vi "Linear Brass25 Calculations.vi"(0 "Power":dbl, 2 "Diameter":dbl, 3 "X1":dbl[](array[numeric]), 5 "T1":dbl[](array[numeric]), 6 "X2":dbl[](array[numeric]), 10 "T2":dbl[](array[numeric]), 11 "X3":dbl[](array[numeric]), 12 "T3":dbl[](array[numeric])) -> (16 "K1-2":dbl, 17 "K2-3":dbl, 18 "K3-4":dbl, 19 "K4-5":dbl, 20 "XY Graph":cluster{"Ramp Pattern":dbl[], dbl[]}[](graph), 21 "K5-6":dbl, 22 "K6-7":dbl, 23 "K7-8":dbl)   [LabVIEW 2017]
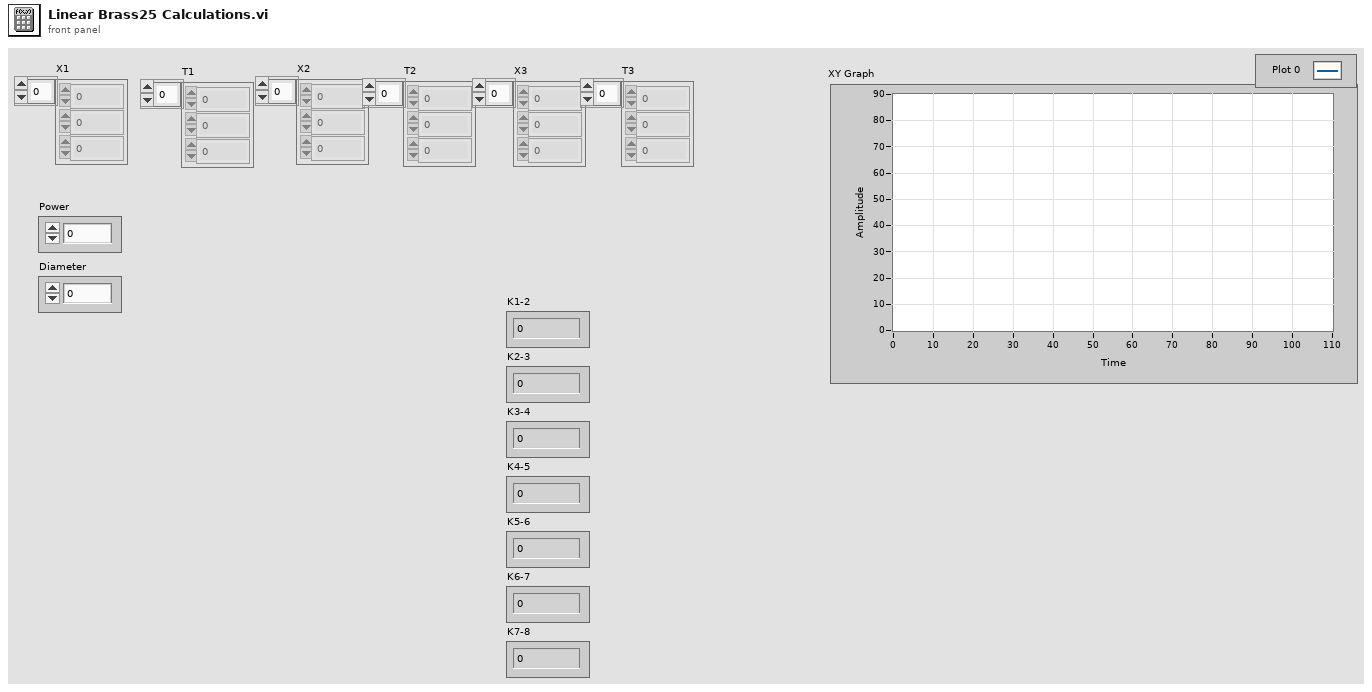
[diagram p1: front panel]
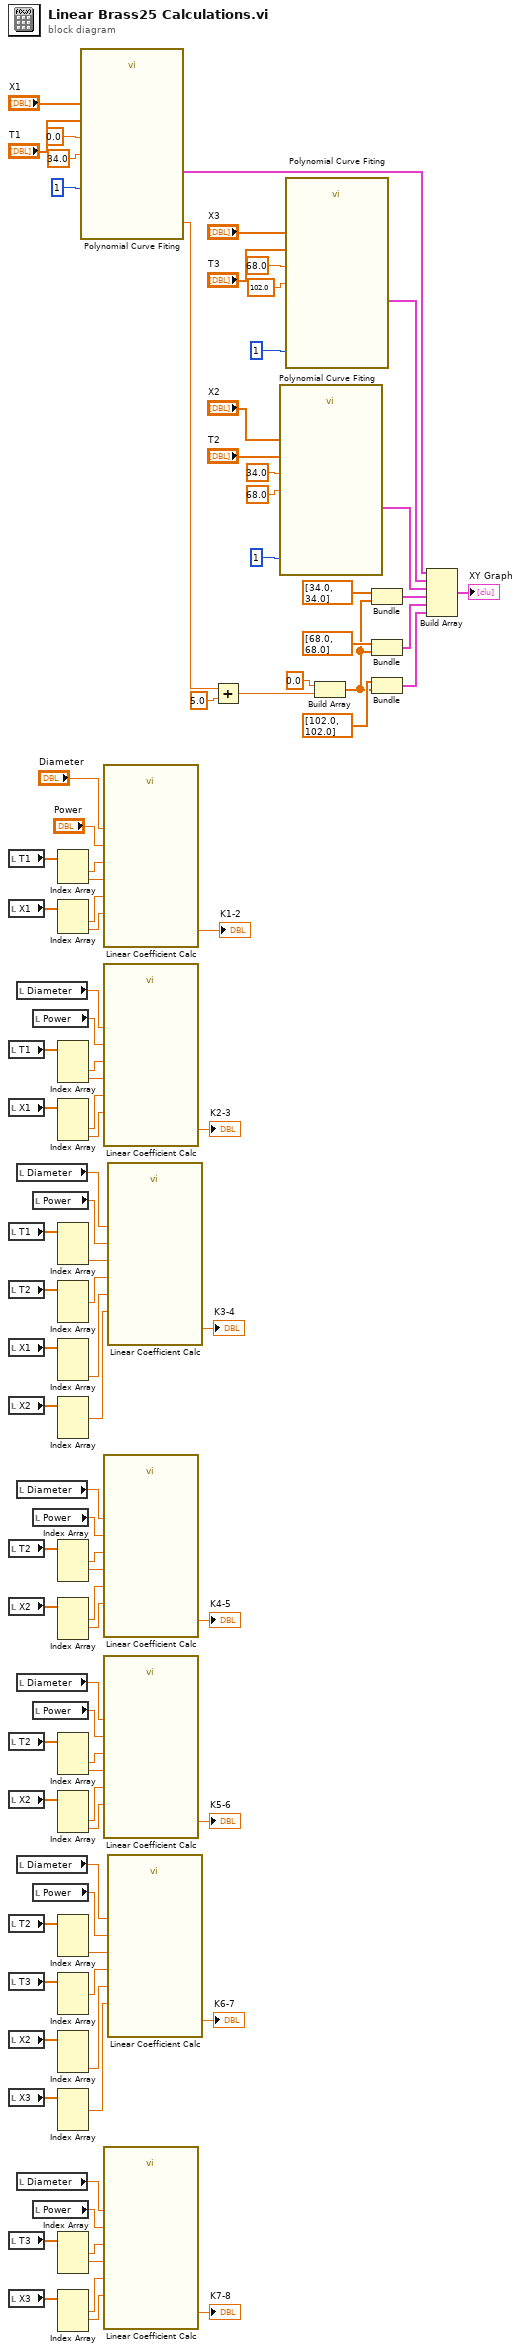
[diagram p0: block diagram]
diagram:
  n1 = local read "T1"() -> (w65:dbl[])
  n2 = local read "X1"() -> (w64:dbl[])
  n3 = local read "T1"() -> (w56:dbl[])
  n4 = local read "X1"() -> (w57:dbl[])
  n5 = local read "T1"() -> (w49:dbl[])
  n6 = local read "T2"() -> (w43:dbl[])
  n7 = local read "X1"() -> (w48:dbl[])
  n8 = local read "X2"() -> (w41:dbl[])
  n9 = local read "T2"() -> (w11:dbl[])
  n10 = local read "X2"() -> (w12:dbl[])
  n11 = local read "T2"() -> (w34:dbl[])
  n12 = local read "X2"() -> (w33:dbl[])
  n13 = local read "T2"() -> (w21:dbl[])
  n14 = local read "T3"() -> (w27:dbl[])
  n15 = local read "X2"() -> (w22:dbl[])
  n16 = local read "X3"() -> (w29:dbl[])
  n17 = local read "T3"() -> (w16:dbl[])
  n18 = local read "X3"() -> (w17:dbl[])
  n19 = local read "Diameter"() -> (w60:dbl)
  n20 = local read "Diameter"() -> (w46:dbl)
  n21 = local read "Diameter"() -> (w14:dbl)
  n22 = local read "Diameter"() -> (w31:dbl)
  n23 = local read "Diameter"() -> (w24:dbl)
  n24 = local read "Diameter"() -> (w19:dbl)
  n25 = local read "Power"() -> (w59:dbl)
  n26 = local read "Power"() -> (w47:dbl)
  n27 = local read "Power"() -> (w13:dbl)
  n28 = local read "Power"() -> (w32:dbl)
  n29 = local read "Power"() -> (w23:dbl)
  n30 = local read "Power"() -> (w18:dbl)
  n31 = Index Array(array=w65) -> (element #1=w63:dbl, element #2=w62:dbl)  [unwired: 2 in]
  n32 = Index Array(array=w64) -> (element #1=w61:dbl, element #2=w58:dbl)  [unwired: 2 in]
  n33 = Index Array(array=w56) -> (element #2=w55:dbl, element #3=w54:dbl)  [unwired: 3 in, 1 out]
  n34 = Index Array(array=w57) -> (element #2=w53:dbl, element #3=w52:dbl)  [unwired: 3 in, 1 out]
  n35 = Index Array(array=w49) -> (element #3=w45:dbl)  [unwired: 3 in, 2 out]
  n36 = Index Array(array=w43) -> (element #1=w42:dbl)  [unwired: 3 in, 2 out]
  n37 = Index Array(array=w48) -> (element #3=w44:dbl)  [unwired: 3 in, 2 out]
  n38 = Index Array(array=w41) -> (element #1=w40:dbl)  [unwired: 3 in, 2 out]
  n39 = Index Array(array=w11) -> (element #1=w9:dbl, element #2=w8:dbl)  [unwired: 3 in, 1 out]
  n40 = Index Array(array=w12) -> (element #1=w7:dbl, element #2=w6:dbl)  [unwired: 3 in, 1 out]
  n41 = Index Array(array=w34) -> (element #2=w35:dbl, element #3=w36:dbl)  [unwired: 3 in, 1 out]
  n42 = Index Array(array=w33) -> (element #2=w37:dbl, element #3=w38:dbl)  [unwired: 3 in, 1 out]
  n43 = Index Array(array=w21) -> (element #3=w25:dbl)  [unwired: 3 in, 2 out]
  n44 = Index Array(array=w27) -> (element #1=w28:dbl)  [unwired: 3 in, 2 out]
  n45 = Index Array(array=w22) -> (element #3=w26:dbl)  [unwired: 3 in, 2 out]
  n46 = Index Array(array=w29) -> (element #1=w30:dbl)  [unwired: 3 in, 2 out]
  n47 = Index Array(array=w16) -> (element #1=w5:dbl, element #2=w4:dbl)  [unwired: 3 in, 1 out]
  n48 = Index Array(array=w17) -> (element #1=w3:dbl, element #2=w2:dbl)  [unwired: 3 in, 1 out]
  n49 = call "Polynomial Curve Fiting.vi"("polynomial order"=1, "end"=34.0, "start"=0.0, "Y"="T1", "X"="X1") -> ("T First"=w71:dbl, "XY Graph"=w83:cluster{"Ramp Pattern":dbl[], dbl[]})  [unwired: 1 out]
  n50 = call "Linear Coefficient Calc.vi"("Diameter"="Diameter", "Power"="Power", "X2"=w58, "X1"=w61, "T2"=w62, "T1"=w63) -> ("K"=→"K1-2":dbl)
  n51 = call "Linear Coefficient Calc.vi"("Diameter"=w60, "Power"=w59, "X2"=w52, "X1"=w53, "T2"=w54, "T1"=w55) -> ("K"=→"K2-3":dbl)
  n52 = call "Linear Coefficient Calc.vi"("Diameter"=w14, "Power"=w13, "X2"=w6, "X1"=w7, "T2"=w8, "T1"=w9) -> ("K"=→"K4-5":dbl)
  n53 = call "Linear Coefficient Calc.vi"("Diameter"=w31, "Power"=w32, "X2"=w38, "X1"=w37, "T2"=w36, "T1"=w35) -> ("K"=→"K5-6":dbl)
  n54 = call "Linear Coefficient Calc.vi"("Diameter"=w19, "Power"=w18, "X2"=w2, "X1"=w3, "T2"=w4, "T1"=w5) -> ("K"=→"K7-8":dbl)
  n55 = call "Linear Coefficient Calc.vi"("Diameter"=w46, "Power"=w47, "X2"=w40, "X1"=w44, "T2"=w42, "T1"=w45) -> ("K"=→"K3-4":dbl)
  n56 = call "Linear Coefficient Calc.vi"("Diameter"=w24, "Power"=w23, "X2"=w30, "X1"=w26, "T2"=w28, "T1"=w25) -> ("K"=→"K6-7":dbl)
  n57 = Add(x=w71, y=5.0) -> (x+y=w69:dbl)
  n58 = call "Polynomial Curve Fiting.vi"("polynomial order"=1, "end"=68.0, "start"=34.0, "Y"="T2", "X"="X2") -> ("XY Graph"=w81:cluster{"Ramp Pattern":dbl[], dbl[]})  [unwired: 2 out]
  n59 = call "Polynomial Curve Fiting.vi"("polynomial order"=1, "end"=102.0, "start"=68.0, "Y"="T3", "X"="X3") -> ("XY Graph"=w82:cluster{"Ramp Pattern":dbl[], dbl[]})  [unwired: 2 out]
  n60 = Build Array(0.0 ("element"), w69) -> (w73:dbl[])
  n61 = Bundle("X Line 1"=dbl[] [34.0, 34.0], w73) -> (w77:cluster{"X Line 1":dbl[], dbl[]})  [unwired: 1 in]
  n62 = Bundle("X Line 2"=dbl[] [68.0, 68.0], w73) -> (w75:cluster{"X Line 2":dbl[], dbl[]})  [unwired: 1 in]
  n63 = Bundle("X Line 3"=dbl[] [102.0, 102.0], w73) -> (w72:cluster{"X Line 3":dbl[], dbl[]})  [unwired: 1 in]
  n64 = Build Array(w83, w82, w81, w77, w75, w72) -> (→"XY Graph":cluster{"X Line 3":dbl[], dbl[]}[])
